vi "Connect.vi"(8 "error in":errorcluster, 10 "endpoint":string, 11 "socket in":refnum<class "Socket.lvclass">) -> (0 "error out":errorcluster, 3 "socket out":refnum<class "Socket.lvclass">)   [LabVIEW 2025, in "ZeroMQ.lvlib" / "Socket.lvclass"]
doc: "Attempt to connect the socket created with zmq_socket to the given <b>endpoint</b>. The endpoint string should specify the protocol, host and port for the connection, e.g.\n tcp://localhost:1234\n inproc://namedprocess\n\nNote that unlike regular TCP sockets, you can connect to a host without the host having bound the port first.\n\nDetailed API documentation: http://api.zeromq.org/3-2:zmq-connect"
uses:
  Socket.lvclass
  Socket.lvclass/Socket.ctl
  libzmq-v143-mt-4_3_6/LibZMQ.lvlib
panel:
  # "ØMQ"
  # "labview"
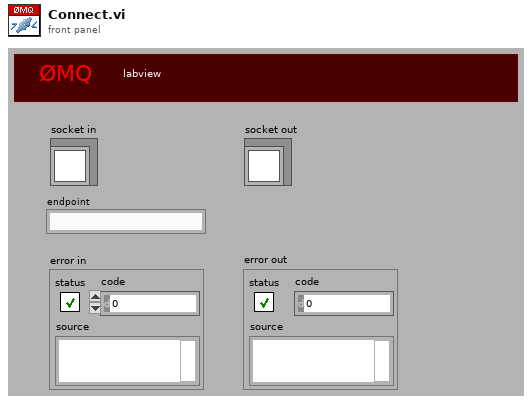
[diagram p1: front panel]
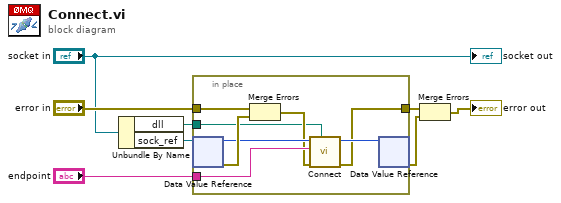
[diagram p0: block diagram]
diagram:
  n1 = Unbundle By Name("socket in") -> ("dll"=w1:path, "sock_ref"=w4:refnum<data-value>)
  n2 = in-place {
    in-place-border: "endpoint" -> [w12]
    in-place-border: "error in" -> [w16]
    in-place-border: [w10] -> w6
    in-place-border: w1 -> [w9]
    n3 = in-place-dvr #1(w4) -> (w14:u64, w15:errorcluster)
    n4 = Merge Errors(w16, w15) -> (w11:errorcluster)
    n5 = call "Connect.vi"("path override"=w9, "error in (no error)"=w11, "addr_"=w12, "s_"=w14) -> ("error out"=w10:errorcluster, "s_ out"=w13:u64)  [unwired: 6 in]
    n6 = in-place-dvr #1(w13) -> (w2:errorcluster)  [unwired: 1 out]
  }
  n7 = Merge Errors(w6, w2) -> (→"error out":errorcluster)
  "socket out" <- "socket in"
